vi "Actor Core.vi"(8 "error in":cluster{"状态":bool, "代码":i32, "源":string} caption="错误输入", 11 "定时循环控制器":refnum<class "Timed Loop Actor.lvclass">) -> (0 "error out":cluster{"状态":bool, "代码":i32, "源":string} caption="错误输出", 3 "操作者输出":refnum<class "Actor.lvclass">)   [LabVIEW 2015, in "Timed Loop Actor.lvlib" / "Timed Loop Actor.lvclass"]
doc: "Actor Core.vi包含操作者的主要消息处理循环。操作者通常位于该循环中，在各种消息到达时对消息进行处理。如Do.vi消息返回任何错误，该循环将停止运行，错误代码43将被作为“无错误停止”的标准信号发送给调用方。如需更改上述行为，可在子孙类的Handle Error.vi中对该部分逻辑进行重写。"
uses:
  Timed Loop Actor.lvclass
  <vilib>/ActorFramework/Actor/Actor.lvclass
  <vilib>/ActorFramework/Actor/Actor.lvclass/Actor.ctl
  <vilib>/ActorFramework/Message Enqueuer/Message Enqueuer.lvclass/Message Enqueuer.ctl
  Timed Loop Actor.lvclass/Timed Loop Actor.ctl
  <vilib>/ActorFramework/Message Enqueuer/Init from Existing Queue.vi
  <vilib>/ActorFramework/Message Enqueuer/Enqueue.vi
  <vilib>/Utility/LVClass/Get LV Class Path.vi
  <vilib>/ActorFramework/Message Priority Queue/Priority Enqueue.vi
  <vilib>/ActorFramework/Message Enqueuer/Message Enqueuer.lvclass
  Update Msg/Update Msg.lvclass
  <vilib>/Platform/TimedLoop/XDataNode/XDataNode.xnode
  <vilib>/Platform/TimedLoop/XDataNode/timing_clust.ctl
  <vilib>/Platform/TimedLoop/XDataNode/XDNodeRunTimeDep.lvlib
  <vilib>/Platform/TimedLoop/XDataNode/wakeup.ctl
  <vilib>/Platform/TimedLoop/XDataNode/nitl_modes.ctl
panel:
  in  "停止？":bool
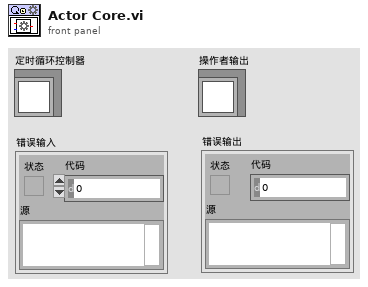
[diagram p1: front panel]
types:
  T1 = typedef "XDNodeRunTimeDep.lvlib/timing_clust.ctl" = cluster{"Expected End [f-1]":u64, "Actual End [f-1]":u64, "Finished Late? [f-1]":bool, "Expected End [i-1]":u64, "Actual End [i-1]":u64, "Finished Late? [i-1]":bool, "Expected Start [i]":u64, "Actual Start [i]":u64, "Expected Start [f]":u64, "Actual Start [f]":u64, "Source Name":string, "Structure Name":string, "Period":i64, "Deadline":i64, "Offset":i64, "Start":i64, "Priority":i32, "Timeout":i32, "Mode":T2, "Wakeup Reason":T3, "Error":errorcluster, "Source Type":string, "Secondary Source Type":string, "Global End Time":u64, "Global Start Time":u64, "Frame Duration":u64, "Iteration Duration":u64, "Assigned CPU":i32, "I/O Scan Engine Mode":u32}
  T2 = typedef "XDNodeRunTimeDep.lvlib/nitl_modes.ctl" = enum32{"No Change", "Process missed periods, maintain original phase", "Discard missed periods, maintain original phase", "Process missed periods, ignore original phase", "Discard missed periods, ignore original phase"}
  T3 = typedef "XDNodeRunTimeDep.lvlib/wakeup.ctl" = enum32{"Normal", "Aborted", "Asynchronous wakeup", "Timing source error", "Timed loop error", "Timeout"}
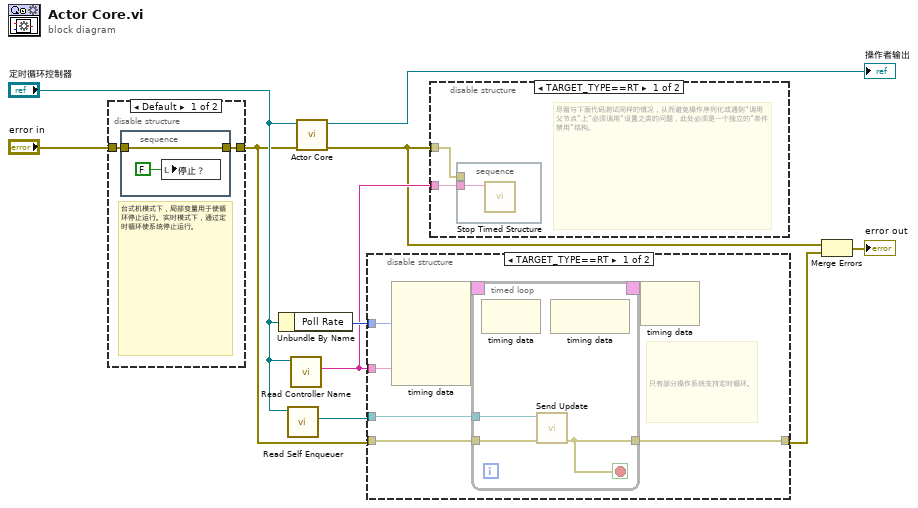
[diagram p0: block diagram]
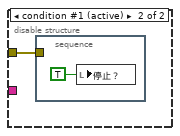
[diagram p3: hidden frame]
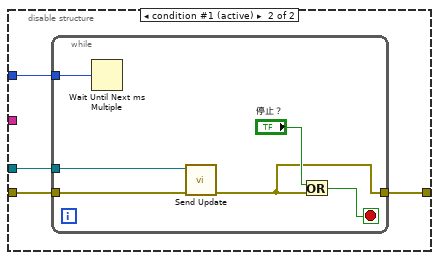
[diagram p4: hidden frame]
diagram:
  n1 = disable-structure shown="Default" {
    disable-tunnel: [w12 _] -> w2
    disable-tunnel: "error in" -> [w11 _]
    frame condition #0 (active) {
      # "台式机模式下，局部变量用于使循环停止运行。实时模式下，通过定时循环使系统停止运行。"
      n2 = stacked-sequence {
        tunnel: [w13] -> w12
        tunnel: w11 -> [w13]
        frame #0 {
          n3 = local write "停止？"(FALSE) -> ()
        }
      }
    }
    frame condition #1 {
    }
  }
  n4 = Unbundle By Name("定时循环控制器") -> ("Poll Rate"=w9:i64)
  n5 = call <vilib>:"Read Self Enqueuer.vi"("Actor"="定时循环控制器") -> ("Self Enqueuer"=w10:refnum<class "Message Enqueuer.lvclass">)  [unwired: 10 in]
  n6 = call "Read Controller Name.vi"("定时循环控制器"="定时循环控制器") -> ("控制器名称"=w7:string)  [unwired: 10 in]
  n7 = call-parent "Actor Core.vi"("error in"=w2, "Actor in"="定时循环控制器") -> ("error out"=w5:errorcluster, "Actor out"=→"操作者输出":refnum<class "Actor.lvclass">)  [unwired: 8 in]
  n8 = disable-structure shown="TARGET_TYPE==RT" {
    disable-tunnel: w10 -> [w19 w35]
    disable-tunnel: w9 -> [w18 w34]
    disable-tunnel: w7 -> [w17 _]
    disable-tunnel: w2 -> [w16 w33]
    disable-tunnel: [w15 w32] -> w4
    frame condition #0 {
      # "只有部分操作系统支持定时循环。"
      n9 = node-c288(w18, w17) -> (w21:T1)  [unwired: 3 in]
      n10 = timed-loop {
        timing: w21 -> [_]
        timing-out: [_] -> w20
        tunnel: w19 -> [w24]
        tunnel: w16 -> [w23]
        tunnel: [w22] -> w15
        stop <- w22 stop-if-true
        n11 = node-c288() -> ()  [unwired: 1 in, 1 out]
        n12 = call "Send Update.vi"("error in (no error)"=w23, "消息待入队列"=w24) -> ("error out"=w22:cluster{"状态":bool, "代码":i32, "源":string})  [unwired: 9 in]
        n13 = node-c288() -> ()  [unwired: 1 in, 1 out]
      }
      n14 = node-c288(w20) -> ()  [unwired: 1 out]
    }
    frame condition #1 (active) {
      n15 = while {
        tunnel: w35 -> [w41]
        tunnel: w34 -> [w40]
        tunnel: w33 -> [w39]
        tunnel: [w36] -> w32
        stop <- w37 stop-if-true
        n16 = Wait Until Next ms Multiple(millisecond multiple=w40) -> ()  [unwired: 1 out]
        n17 = call "Send Update.vi"("error in (no error)"=w39, "消息待入队列"=w41) -> ("error out"=w36:cluster{"状态":bool, "代码":i32, "源":string})  [unwired: 9 in]
        n18 = Or(x="停止？", y=w36) -> (x .or. y?=w37:bool)
      }
    }
  }
  n19 = disable-structure shown="TARGET_TYPE==RT" {
    disable-tunnel: w5 -> [w42 w45]
    disable-tunnel: w7 -> [w43 _]
    frame condition #0 {
      # "尽管与下面代码测试同样的情况，从而避免操作序列化或遇到“调用父节点”上“必须调用”设置之类的问题，此处必须是一个独立的“条件禁用”结构。"
      n20 = stacked-sequence {
        tunnel: w43 -> [w44]
        tunnel: w42 -> [_]
        frame #0 {
          n21 = call <vilib>:"Stop Timed Structure.vi"("name"=w44) -> ()  [unwired: 10 in, 1 out]
        }
      }
    }
    frame condition #1 (active) {
      n22 = stacked-sequence {
        tunnel: w45 -> [_]
        frame #0 {
          n23 = local write "停止？"(TRUE) -> ()
        }
      }
    }
  }
  n24 = Merge Errors(w5, w4) -> (→"error out":errorcluster)
